vi "Scanner Queue - Get.vi"(8 "error in":errorcluster) -> (0 "error out":errorcluster, 3 "queue out":refnum<queue>)   [LabVIEW 2024, in "Session Scanner.lvlib"]
uses:
  Session Scanner.lvlib
  Support/General Type Defs/Queue Message.ctl
  Support/General Type Defs/FGV States.ctl
  Support/General Type Defs/General Type Defs.lvlib
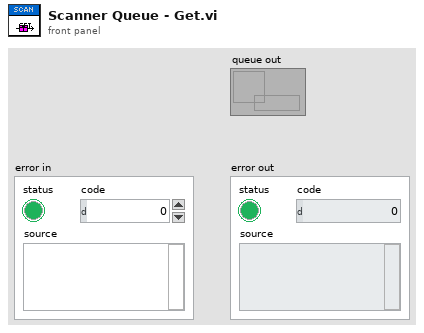
[diagram p1: front panel]
types:
  T1 = typedef "General Type Defs.lvlib/FGV States.ctl" = enum16{"Create", "Get", "Destroy"}
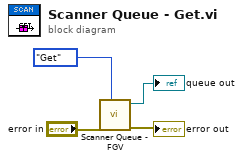
[diagram p0: block diagram]
diagram:
  n1 = call "Scanner Queue - FGV.vi"("FGV States"=FGV_States."Get", "error in"="error in") -> ("error out"=→"error out":errorcluster, "queue out"=→"queue out":refnum<queue>)  [unwired: 8 in]
